vi "TDMS Cleanup.vi"(0 "Logging in":refnum<class "Logging.lvclass">, 1 "Task Selection":T2={"Task Type Select"=enum."Frequency Task", "Input Select Type"=enum."Force Input", "Collect EMG?"=FALSE, "Collect acceleration?"=FALSE, "EMG Rate"=200, "Acceleration Rate"=200} {"Acceleration Rate" min=1 step=1; "EMG Rate" min=1 step=1}, 2 "Task info":T3={"Number of Trials"=1, "Sampling Rate (Hz)"=200, "Trial Duration (s)"=10, "Adjusted MVC (N)"=5.0, "R Phase"=0, "L Phase"=0, "L Pattern"=1, "R Pattern"=1, "Time Between Trials (s)"=5, "Lissajous Speed"=200} {"Lissajous Speed" min=1 max=200; "Time Between Trials (s)" min=1 step=1; "R Pattern" min=1 max=20 step=1; "L Pattern" min=1 max=20 step=1; "L Phase" min=-180 max=180 step=1; "R Phase" min=-180 max=180 step=1; "Adjusted MVC (N)" min=1.0 max=50.0 step=0.10000000149011612; "Trial Duration (s)" min=1 step=1; "Sampling Rate (Hz)" min=1 step=1; "Number of Trials" min=1 step=1}, 5 "TDMS File":path, 7 "Accel TDMS File":refnum<k34>, 9 "Force TDMS File":refnum<k34>, 11 "error in (no error)":errorcluster, 12 "Movement?":bool, 13 "Auto Clust":T1={"Automate?"=FALSE, "Num Parabs"=1, "Patterns Array"=[], "Phase Array"=[]} {"Num Parabs" min=1 step=1}) -> (4 "Logging out":refnum<class "Logging.lvclass">, 15 "error out":errorcluster)   [LabVIEW 2020, in "Logging.lvlib" / "Logging.lvclass"]
uses:
  Logging.lvclass
  C:/Program Files/National Instruments/LabVIEW 2020/vi.lib/ActorFramework/Actor/Actor.lvclass
  Task info df.ctl
  Task selection df.ctl
  Automate df.ctl
  <vilib>/ActorFramework/Actor/Actor.lvclass/Actor.ctl
  <vilib>/ActorFramework/Message Enqueuer/Message Enqueuer.lvclass/Message Enqueuer.ctl
  Logging.lvclass/Logging.ctl
  <vilib>/ActorFramework/Message Enqueuer/Init from Existing Queue.vi
  <vilib>/Utility/file.llb/Read Delimited Spreadsheet (DBL).vi
  <vilib>/ActorFramework/Message Enqueuer/Message Enqueuer.lvclass
  Logging Messages/Convert to Excel Msg/Convert to Excel Msg.lvclass
  <vilib>/ActorFramework/Actor/Actor.lvclass
panel:
  # "Patterns"
  # "Phase"
  # "Left        Right"
  # "Left        Right"
  # "Input Type"
  # "Task Type"
  # "Left Arm"
  # "Right Arm"
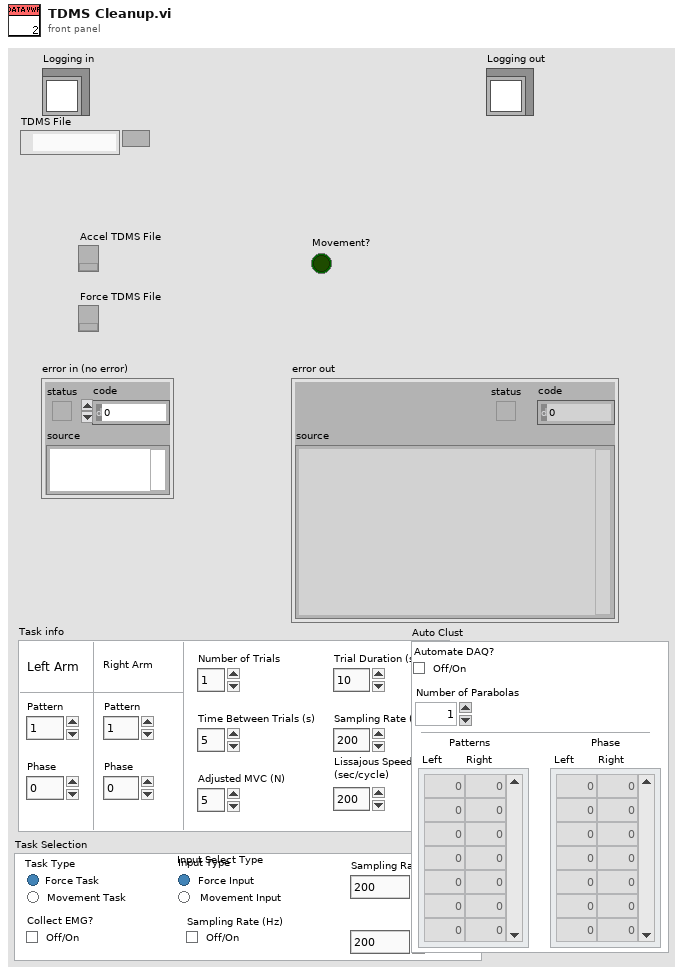
[diagram p1: front panel]
types:
  T1 = typedef "Automate df.ctl" = cluster{"Automate?":bool, "Num Parabs":u16, "Patterns Array":u8[][], "Phase Array":i32[][]}
  T2 = typedef "Task selection df.ctl" = cluster{"Task Type Select":enum32{"Frequency Task", "Scanning Task"}, "Input Select Type":enum32{"Force Input", "Movement Input"}, "Collect EMG?":bool, "Collect acceleration?":bool, "EMG Rate":u16, "Acceleration Rate":u16}
  T3 = typedef "Task info df.ctl" = cluster{"Number of Trials":u8, "Sampling Rate (Hz)":u16, "Trial Duration (s)":u8, "Adjusted MVC (N)":dbl, "R Phase":i32, "L Phase":i32, "L Pattern":u8, "R Pattern":u8, "Time Between Trials (s)":u8, "Lissajous Speed":u16}
  T4 = enum16{"open", "open or create", "create or replace", "create", "open (read-only)"}
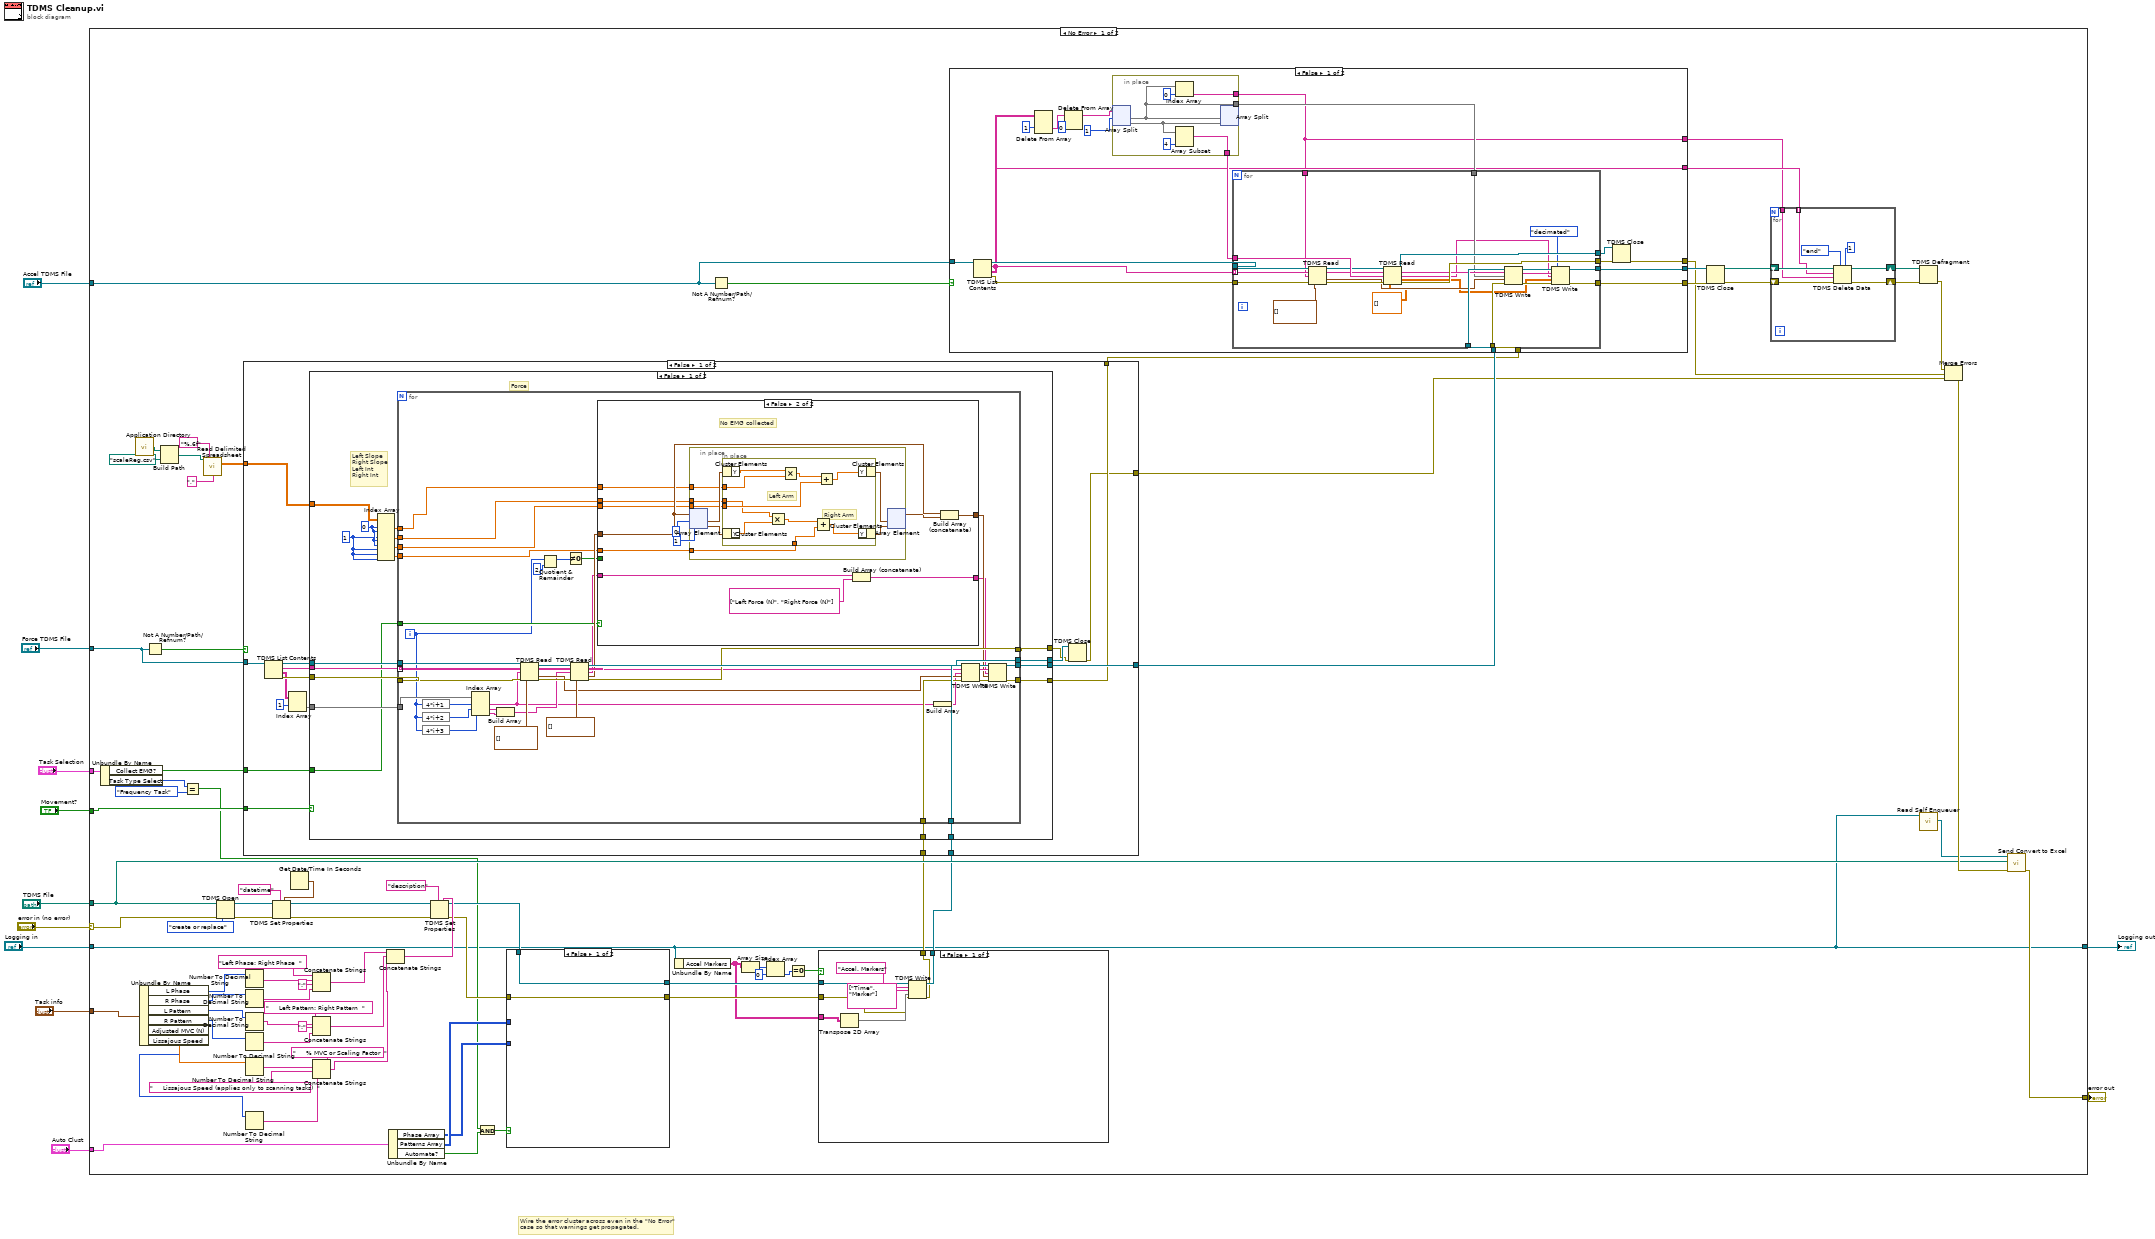
[diagram p0: block diagram]
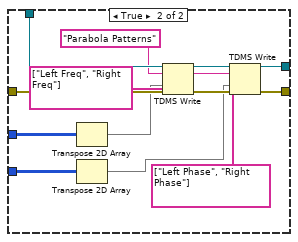
[diagram p3: hidden frame]
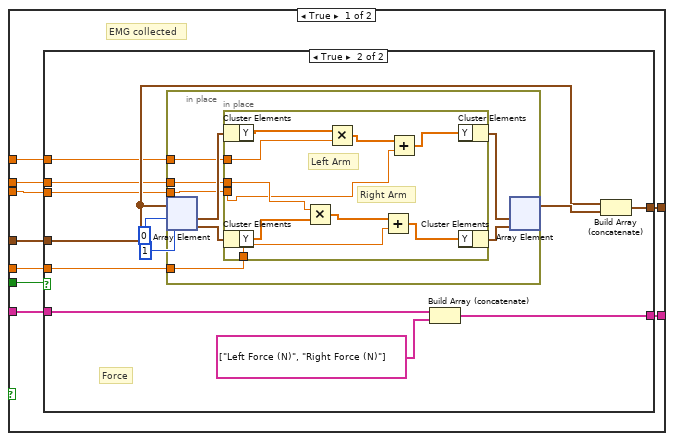
[diagram p4: hidden frame]
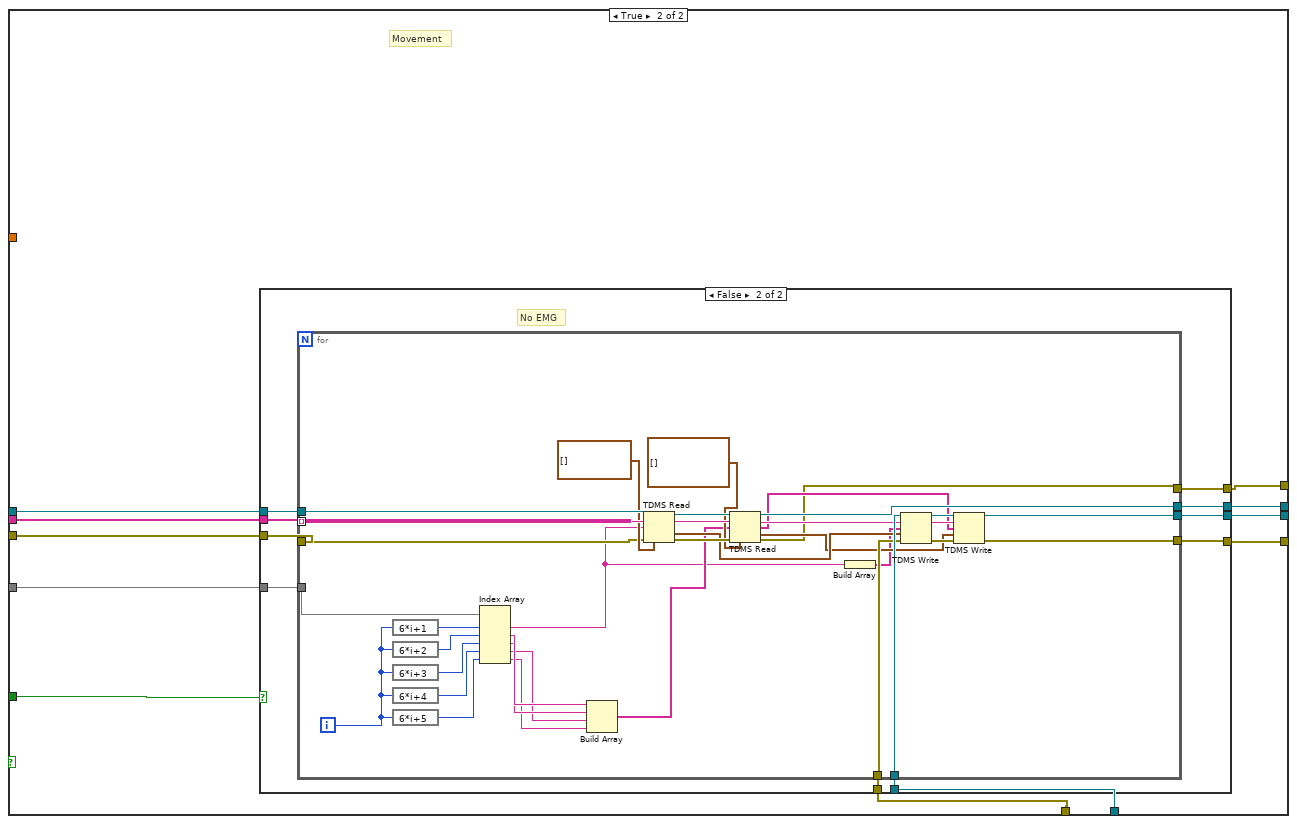
[diagram p6: hidden frame]
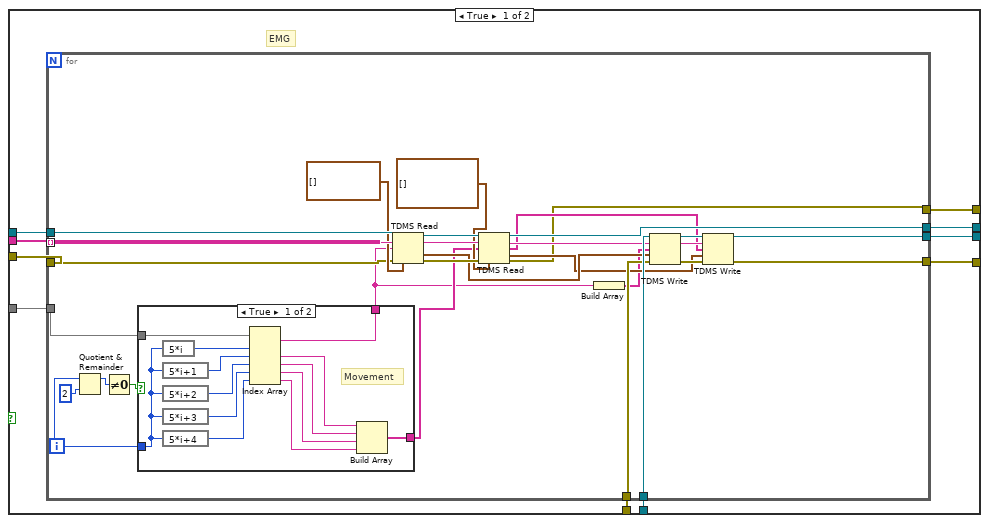
[diagram p7: hidden frame]
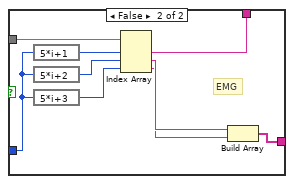
[diagram p8: hidden frame]
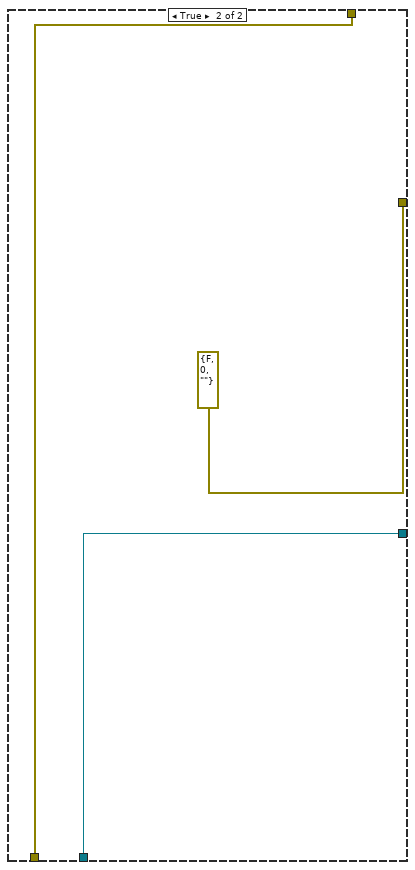
[diagram p9: hidden frame]
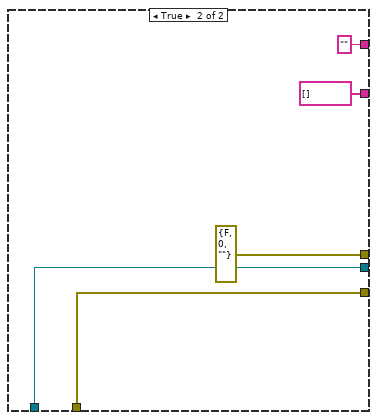
[diagram p10: hidden frame]
diagram:
  # "Wire the error cluster across even in the \"No Error\"\ncase so that warnings get propagated."
  n1 = case shown="No Error" "error in (no error)" {
    selector: "error in (no error)" -> [w82 w452]
    tunnel: [w45 w452] -> w10
    tunnel: [w24 w451] -> w8
    tunnel: "Logging in" -> [w24 w451]
    tunnel: "Accel TDMS File" -> [w85 _]
    tunnel: "Force TDMS File" -> [w86 _]
    tunnel: "TDMS File" -> [w46 _]
    tunnel: "Movement?" -> [w76 _]
    tunnel: "Task Selection" -> [w75 _]
    tunnel: "Task info" -> [w72 _]
    tunnel: "Auto Clust" -> [w43 _]
    frame No Error {
      n2 = Unbundle By Name(w75) -> ("Collect EMG?"=w74:bool, "Task Type Select"=w29:enum32{"Frequency Task", "Scanning Task"})
      n3 = call <vilib>:"Application Directory.vi"() -> ("Application Directory"=w22:path)
      n4 = Unbundle By Name(w72) -> ("L Phase"=w71:i32, "R Phase"=w70:i32, "L Pattern"=w69:u8, "R Pattern"=w68:u8, "Adjusted MVC (N)"=w67:dbl, "Lissajous Speed"=w56:u16)
      n5 = Not A Number/Path/Refnum?(number/path/refnum=w86) -> (NaN/Path/Refnum?=w87:bool)
      n6 = Build Path(base path=w22, name or relative path=path "scaleReg.csv") -> (appended path=w23:path)
      n7 = Equal?(x=w29, y=enum32{"Frequency Task", "Scanning Task"}."Frequency Task") -> (x = y?=w25:bool)
      n8 = call-poly <vilib>:"Read Delimited Spreadsheet.vi"("file path (dialog if empty)"=w23, "format (%.3f)"="%.6f", "delimiter (\\t)"="," ("delimiter (\\t)")) -> ("all rows"=w18:dbl[][])  [unwired: 7 in, 5 out]
      n9 = TDMS Open(8:w82, 10:T4."create or replace" ("operation (0:open)"), 11:w46) -> (0:w91:errorcluster, 3:w92:refnum<k34>)  [unwired: 4 in]
      n10 = Number To Decimal String(number=w71) -> (decimal integer string=w65:string)  [unwired: 1 in]
      n11 = Number To Decimal String(number=w70) -> (decimal integer string=w58:string)  [unwired: 1 in]
      n12 = Number To Decimal String(number=w69) -> (decimal integer string=w64:string)  [unwired: 1 in]
      n13 = Number To Decimal String(number=w68) -> (decimal integer string=w61:string)  [unwired: 1 in]
      n14 = Number To Decimal String(number=w67) -> (decimal integer string=w59:string)  [unwired: 1 in]
      n15 = Number To Decimal String(number=w56) -> (decimal integer string=w55:string)  [unwired: 1 in]
      n16 = Get Date/Time In Seconds() -> (seconds since 1Jan1904=w89:timestamp)
      n17 = TDMS Set Properties(5:w89, 7:"datetime", 8:w91, 11:w92) -> (0:w49:errorcluster, 3:w73:refnum<k34>)  [unwired: 2 in, 2 out]
      n18 = Concatenate Strings("Left Phase: Right Phase  " ("string"), w65, ":" ("string"), w58) -> (w54:string)
      n19 = Concatenate Strings("     Left Pattern: Right Pattern  " ("string"), w64, ":" ("string"), w61) -> (w53:string)
      n20 = Concatenate Strings("     % MVC or Scaling Factor  " ("string"), w59, "     Lissajous Speed (applies only to scanning tasks)  " ("string"), w55) -> (w52:string)
      n21 = Concatenate Strings(w54, w53, w52) -> (w51:string)
      n22 = Unbundle By Name(w43) -> ("Phase Array"=w30:i32[][], "Patterns Array"=w42:u8[][], "Automate?"=w26:bool)
      n23 = TDMS Set Properties(5:w51, 7:"description" ("property names"), 8:w49, 11:w73) -> (0:w40:errorcluster, 3:w41:refnum<k34>)  [unwired: 2 in, 2 out]
      n24 = And(x=w25, y=w26) -> (x .and. y?=w27:bool)
      n25 = case shown="False" w27 {
        tunnel: w42 -> [_ w123]
        tunnel: w41 -> [w113 w127]
        tunnel: w40 -> [w112 w126]
        tunnel: [w113 w121] -> w39
        tunnel: [w112 w119] -> w38
        tunnel: w30 -> [_ w115]
        frame False {
        }
        frame True {
          n26 = Transpose 2D Array(2D array=w123) -> (transposed array=w122:u8[][])
          n27 = Transpose 2D Array(2D array=w115) -> (transposed array=w114:i32[][])
          n28 = TDMS Write(0:w127, 5:"Parabola Patterns" ("group name in (Untitled)"), 7:string[] ["Left Freq", "Right Freq"] ("array"), 9:w122, 11:w126) -> (4:w120:refnum<k34>, 6:w117:string, 15:w118:errorcluster)  [unwired: 1 in, 1 out]
          n29 = TDMS Write(0:w120, 5:w117, 7:string[] ["Left Phase", "Right Phase"] ("channel name(s) in (Untitled)"), 9:w114, 11:w118) -> (4:w121:refnum<k34>, 15:w119:errorcluster)  [unwired: 1 in, 2 out]
        }
      }
      n30 = Unbundle By Name(w24) -> ("Accel Markers"=w31:string[][])
      n31 = Not A Number/Path/Refnum?(number/path/refnum=w85) -> (NaN/Path/Refnum?=w88:bool)
      n32 = Array Size(array=w31) -> (size(s)=w37:i32[])
      n33 = Index Array(array=w37, index=0) -> (element=w35:i32)
      n34 = Equal To 0?(x=w35) -> (x = 0?=w34:bool)
      n35 = case shown="False" w34 {
        tunnel: w39 -> [w109 w111]
        tunnel: w38 -> [w102 w110]
        tunnel: [w106 w111] -> w33
        tunnel: [w105 w110] -> w32
        tunnel: w31 -> [w104 _]
        frame False {
          n36 = Transpose 2D Array(2D array=w104) -> (transposed array=w103:string[][])
          n37 = TDMS Write(0:w109, 5:"Accel. Markers" ("group name in (Untitled)"), 7:string[] ["Time", "Marker"] ("channel name(s) in (Untitled)"), 9:w103, 11:w102) -> (4:w106:refnum<k34>, 15:w105:errorcluster)  [unwired: 1 in, 2 out]
        }
        frame True {
        }
      }
      n38 = case shown="False" w87 {
        tunnel: w86 -> [w144 _]
        tunnel: w33 -> [w142 w394]
        tunnel: [w141 w394] -> w84
        tunnel: w32 -> [w140 w393]
        tunnel: [w139 w393] -> w81
        tunnel: [w138 errorcluster {"status"=FALSE, "code"=0, "source"=""} ("error out")] -> w79
        tunnel: w76 -> [w130 _]
        tunnel: w74 -> [w129 _]
        tunnel: w18 -> [w128 _]
        frame False {
          n39 = TDMS List Contents(7:w144) -> (0:w134:errorcluster, 1:w133:string[][], 2:w137:string[], 3:w143:refnum<k34>)  [unwired: 2 in]
          n40 = Index Array(array=w133, index (row)=1) -> (element=w131:string[])  [unwired: 1 in]
          n41 = case shown="False" w130 {
            tunnel: w143 -> [w162 w285]
            tunnel: w142 -> [w161 w284]
            tunnel: [w160 w283] -> w141
            tunnel: w140 -> [w159 w282]
            tunnel: [w158 w281] -> w139
            tunnel: w137 -> [w157 w280]
            tunnel: [w156 w279] -> w136
            tunnel: [w155 w278] -> w135
            tunnel: w134 -> [w154 w277]
            tunnel: w131 -> [w153 w276]
            tunnel: w129 -> [w152 w275]
            tunnel: w128 -> [w145 _]
            frame False {
              w150 = 1 ("index (row)")
              w151 = 0 ("index (row)")
              # "Left Slope\nRight Slope\nLeft Int\nRight Int"
              # "Force"
              n42 = Index Array(array=w145, index (row) #1=w151, index (col) #1=w151, index (row) #2=w150, index (col) #2=w151, index (row) #3=w151, index (col) #3=w150, index (row) #4=w150, index (col) #4=w150) -> (element #1=w149:dbl, element #2=w147:dbl, element #3=w148:dbl, element #4=w146:dbl)
              n43 = for {
                tunnel: w162 -> [w203]
                tunnel: w157 -> [w202] mode=indexing
                tunnel: w161 -> [w201]
                tunnel: [w193] -> w160
                tunnel: w159 -> [w200]
                tunnel: [w190] -> w158
                tunnel: [w198] -> w156
                tunnel: [w187] -> w155
                tunnel: w154 -> [w186]
                tunnel: w153 -> [w185]
                tunnel: w152 -> [w174]
                tunnel: w149 -> [w166]
                tunnel: w148 -> [w165]
                tunnel: w147 -> [w164]
                tunnel: w146 -> [w163]
                i -> [w173]
                n44 = expression code="4*i+1"(w173) -> (w184:i32)
                n45 = expression code="4*i+2"(w173) -> (w183:i32)
                n46 = expression code="4*i+3"(w173) -> (w182:i32)
                n47 = Index Array(array=w185, index #1=w184, index #2=w183, index #3=w182) -> (element #1=w178:string, element #2=w181:string, element #3=w180:string)
                n48 = Build Array(w181, w180) -> (w179:string[])
                n49 = TDMS Read(0:w203, 5:w202, 7:w178, 11:w186, 12:timestamp[] []) -> (4:w199:refnum<k34>, 6:w197:string, 10:w188:timestamp[], 15:w196:errorcluster)  [unwired: 3 in, 2 out]
                n50 = Quotient & Remainder(x=w173, y=2) -> (x-y*floor(x/y)=w171:i32)  [unwired: 1 out]
                n51 = Not Equal To 0?(x=w171) -> (x != 0?=w170:bool)
                n52 = TDMS Read(0:w199, 5:w197, 7:w179, 11:w196, 12:waveform(dbl)[] [] ("data")) -> (4:w198:refnum<k34>, 6:w167:string, 8:w169:string[], 10:w176:waveform(dbl)[], 15:w187:errorcluster)  [unwired: 3 in, 1 out]
                n53 = case shown="False" w174 {
                  tunnel: w176 -> [w211 w255]
                  tunnel: [w212 w256] -> w175
                  tunnel: w170 -> [w210 _]
                  tunnel: w169 -> [w209 w250]
                  tunnel: [w208 w249] -> w168
                  tunnel: w166 -> [w207 w248]
                  tunnel: w165 -> [w205 w247]
                  tunnel: w164 -> [w206 w246]
                  tunnel: w163 -> [w204 w245]
                  frame True {
                    # "EMG collected"
                    n54 = case shown="True" w210 {
                      tunnel: [w214 w223] -> w212
                      tunnel: w211 -> [w214 w222]
                      tunnel: w209 -> [w213 w221]
                      tunnel: [w213 w219] -> w208
                      tunnel: w207 -> [_ w218]
                      tunnel: w206 -> [_ w217]
                      tunnel: w205 -> [_ w216]
                      tunnel: w204 -> [_ w215]
                      frame False {
                        # "EMG"
                      }
                      frame True {
                        # "Force"
                        n55 = in-place {
                          in-place-border: w218 -> [w230]
                          in-place-border: w217 -> [w229]
                          in-place-border: w216 -> [w228]
                          in-place-border: w215 -> [w227]
                          n56 = in-place-array #1(w222, 0, 1) -> (w234:waveform(dbl), w233:waveform(dbl))
                          n57 = in-place {
                            in-place-border: w230 -> [w238]
                            in-place-border: w229 -> [w237]
                            in-place-border: w228 -> [w236]
                            in-place-border: w227 -> [w235]
                            # "Right Arm"
                            # "Left Arm"
                            n58 = in-place-cluster #2(w234) -> ("Y"=w243:dbl[])
                            n59 = in-place-cluster #3(w233) -> ("Y"=w239:dbl[])
                            n60 = Multiply(x=w237, y=w239) -> (x*y=w241:dbl[])
                            n61 = Multiply(x=w243, y=w238) -> (x*y=w244:dbl[])
                            n62 = Add(x=w241, y=w235) -> (x+y=w240:dbl[])
                            n63 = Add(x=w244, y=w236) -> (x+y=w242:dbl[])
                            n64 = in-place-cluster #2("Y"=w242) -> (w231:waveform(dbl))
                            n65 = in-place-cluster #3("Y"=w240) -> (w232:waveform(dbl))
                          }
                          n66 = in-place-array #1(w231, w232) -> (w224:waveform(dbl)[])  [unwired: 2 out]
                        }
                        n67 = Build Array (concatenate)(w221, string[] ["Left Force (N)", "Right Force (N)"] ("array")) -> (w219:string[])
                        n68 = Build Array (concatenate)(w222, w224) -> (w223:waveform(dbl)[])
                      }
                    }
                  }
                  frame False {
                    # "No EMG collected"
                    n69 = in-place {
                      in-place-border: w248 -> [w260]
                      in-place-border: w247 -> [w259]
                      in-place-border: w246 -> [w258]
                      in-place-border: w245 -> [w257]
                      n70 = in-place-array #4(w255, 0, 1) -> (w264:waveform(dbl), w263:waveform(dbl))
                      n71 = in-place {
                        in-place-border: w260 -> [w268]
                        in-place-border: w259 -> [w267]
                        in-place-border: w258 -> [w266]
                        in-place-border: w257 -> [w265]
                        # "Right Arm"
                        # "Left Arm"
                        n72 = in-place-cluster #5(w264) -> ("Y"=w273:dbl[])
                        n73 = in-place-cluster #6(w263) -> ("Y"=w269:dbl[])
                        n74 = Multiply(x=w266, y=w269) -> (x*y=w271:dbl[])
                        n75 = Multiply(x=w273, y=w268) -> (x*y=w274:dbl[])
                        n76 = Add(x=w271, y=w265) -> (x+y=w270:dbl[])
                        n77 = Add(x=w274, y=w267) -> (x+y=w272:dbl[])
                        n78 = in-place-cluster #5("Y"=w272) -> (w261:waveform(dbl))
                        n79 = in-place-cluster #6("Y"=w270) -> (w262:waveform(dbl))
                      }
                      n80 = in-place-array #4(w261, w262) -> (w252:waveform(dbl)[])  [unwired: 2 out]
                    }
                    n81 = Build Array (concatenate)(w250, string[] ["Left Force (N)", "Right Force (N)"] ("array")) -> (w249:string[])
                    n82 = Build Array (concatenate)(w255, w252) -> (w256:waveform(dbl)[])
                  }
                }
                n83 = Build Array(w178) -> (w177:string[])
                n84 = TDMS Write(0:w201, 5:w167, 7:w177, 9:w188, 11:w200) -> (4:w192:refnum<k34>, 6:w189:string, 15:w191:errorcluster)  [unwired: 1 in, 1 out]
                n85 = TDMS Write(0:w192, 5:w189, 7:w168, 9:w175, 11:w191) -> (4:w193:refnum<k34>, 15:w190:errorcluster)  [unwired: 1 in, 2 out]
              }
            }
            frame True {
              # "Movement"
              n86 = case shown="False" w275 {
                tunnel: w285 -> [w295 w356]
                tunnel: w284 -> [w294 w355]
                tunnel: [w293 w354] -> w283
                tunnel: w282 -> [w292 w353]
                tunnel: [w291 w352] -> w281
                tunnel: w280 -> [w290 w351]
                tunnel: [w289 w350] -> w279
                tunnel: [w288 w349] -> w278
                tunnel: w277 -> [w287 w348]
                tunnel: w276 -> [w286 w347]
                frame True {
                  # "EMG"
                  n87 = for {
                    tunnel: w295 -> [w324]
                    tunnel: w290 -> [w323] mode=indexing
                    tunnel: w294 -> [w322]
                    tunnel: [w314] -> w293
                    tunnel: w292 -> [w321]
                    tunnel: [w311] -> w291
                    tunnel: [w319] -> w289
                    tunnel: [w305] -> w288
                    tunnel: w287 -> [w304]
                    tunnel: w286 -> [w303]
                    i -> [w299]
                    n88 = Quotient & Remainder(x=w299, y=2) -> (x-y*floor(x/y)=w297:i32)  [unwired: 1 out]
                    n89 = Not Equal To 0?(x=w297) -> (x != 0?=w296:bool)
                    n90 = case shown="True" w296 {
                      tunnel: w303 -> [w337 w346]
                      tunnel: [w331 w340] -> w302
                      tunnel: [w330 w339] -> w301
                      tunnel: w299 -> [w329 w338]
                      frame True {
                        # "Movement"
                        n91 = expression code="5*i"(w329) -> (w336:i32)
                        n92 = expression code="5*i+1"(w329) -> (w335:i32)
                        n93 = expression code="5*i+2"(w329) -> (w334:i32)
                        n94 = expression code="5*i+3"(w329) -> (w328:i32)
                        n95 = expression code="5*i+4"(w329) -> (w327:i32)
                        n96 = Index Array(array=w337, index #1=w336, index #2=w335, index #3=w334, index #4=w328, index #5=w327) -> (element #1=w330:string, element #2=w333:string, element #3=w332:string, element #4=w326:string, element #5=w325:string)
                        n97 = Build Array(w333, w332, w326, w325) -> (w331:string[])
                      }
                      frame False {
                        # "EMG"
                        n98 = expression code="5*i+1"(w338) -> (w345:i32)
                        n99 = expression code="5*i+2"(w338) -> (w344:i32)
                        n100 = expression code="5*i+3"(w338) -> (w343:i32)
                        n101 = Index Array(array=w346, index #1=w345, index #2=w344, index #3=w343) -> (element #1=w339:string, element #2=w342:string, element #3=w341:string)
                        n102 = Build Array(w342, w341) -> (w340:string[])
                      }
                    }
                    n103 = TDMS Read(0:w324, 5:w323, 7:w301, 11:w304, 12:timestamp[] []) -> (4:w320:refnum<k34>, 6:w318:string, 10:w307:timestamp[], 15:w317:errorcluster)  [unwired: 3 in, 2 out]
                    n104 = TDMS Read(0:w320, 5:w318, 7:w302, 11:w317, 12:waveform(dbl)[] [] ("data")) -> (4:w319:refnum<k34>, 6:w310:string, 8:w308:string[], 10:w306:waveform(dbl)[], 15:w305:errorcluster)  [unwired: 3 in, 1 out]
                    n105 = Build Array(w301) -> (w300:string[])
                    n106 = TDMS Write(0:w322, 5:w310, 7:w300, 9:w307, 11:w321) -> (4:w313:refnum<k34>, 6:w309:string, 15:w312:errorcluster)  [unwired: 1 in, 1 out]
                    n107 = TDMS Write(0:w313, 5:w309, 7:w308, 9:w306, 11:w312) -> (4:w314:refnum<k34>, 15:w311:errorcluster)  [unwired: 1 in, 2 out]
                  }
                }
                frame False {
                  # "No EMG"
                  n108 = for {
                    tunnel: w356 -> [w391]
                    tunnel: w351 -> [w390] mode=indexing
                    tunnel: w355 -> [w389]
                    tunnel: [w381] -> w354
                    tunnel: w353 -> [w388]
                    tunnel: [w378] -> w352
                    tunnel: [w386] -> w350
                    tunnel: [w372] -> w349
                    tunnel: w348 -> [w371]
                    tunnel: w347 -> [w370]
                    i -> [w361]
                    n109 = expression code="6*i+1"(w361) -> (w369:i32)
                    n110 = expression code="6*i+2"(w361) -> (w368:i32)
                    n111 = expression code="6*i+3"(w361) -> (w367:i32)
                    n112 = expression code="6*i+4"(w361) -> (w360:i32)
                    n113 = expression code="6*i+5"(w361) -> (w359:i32)
                    n114 = Index Array(array=w370, index #1=w369, index #2=w368, index #3=w367, index #4=w360, index #5=w359) -> (element #1=w363:string, element #2=w366:string, element #3=w365:string, element #4=w358:string, element #5=w357:string)
                    n115 = Build Array(w366, w365, w358, w357) -> (w364:string[])
                    n116 = TDMS Read(0:w391, 5:w390, 7:w363, 11:w371, 12:timestamp[] []) -> (4:w387:refnum<k34>, 6:w385:string, 10:w374:timestamp[], 15:w384:errorcluster)  [unwired: 3 in, 2 out]
                    n117 = TDMS Read(0:w387, 5:w385, 7:w364, 11:w384, 12:waveform(dbl)[] [] ("data")) -> (4:w386:refnum<k34>, 6:w377:string, 8:w375:string[], 10:w373:waveform(dbl)[], 15:w372:errorcluster)  [unwired: 3 in, 1 out]
                    n118 = Build Array(w363) -> (w362:string[])
                    n119 = TDMS Write(0:w389, 5:w377, 7:w362, 9:w374, 11:w388) -> (4:w380:refnum<k34>, 6:w376:string, 15:w379:errorcluster)  [unwired: 1 in, 1 out]
                    n120 = TDMS Write(0:w380, 5:w376, 7:w375, 9:w373, 11:w379) -> (4:w381:refnum<k34>, 15:w378:errorcluster)  [unwired: 1 in, 2 out]
                  }
                }
              }
            }
          }
          n121 = TDMS Close(8:w135, 11:w136) -> (0:w138:errorcluster)  [unwired: 1 out]
        }
        frame True {
        }
      }
      n122 = case shown="False" w88 {
        tunnel: w85 -> [w414 _]
        tunnel: w84 -> [w412 w450]
        tunnel: [w411 w450] -> w83
        tunnel: w81 -> [w409 w449]
        tunnel: [w407 w449] -> w80
        tunnel: [w406 errorcluster {"status"=FALSE, "code"=0, "source"=""} ("error out")] -> w78
        tunnel: [w396 string[] [] ("group names")] -> w13
        tunnel: [w395 ""] -> w12
        frame False {
          n123 = TDMS List Contents(7:w414) -> (0:w397:errorcluster, 1:w402:string[][], 2:w396:string[], 3:w413:refnum<k34>)  [unwired: 2 in]
          n124 = Delete From Array(array=w402, index (row)=1) -> (deleted portion=w404:string[])  [unwired: 2 in, 1 out]
          n125 = Delete From Array(array=w404, index=0) -> (array with subset deleted=w401:string[])  [unwired: 1 in, 1 out]
          n126 = in-place {
            in-place-border: [w415] -> w399
            in-place-border: [w419] -> w395
            in-place-border: [w418] -> w398
            n127 = in-place-split #7(w401, 1) -> (w418:string[], w417:string[])
            n128 = Index Array(array=w418, index=0) -> (element=w419:string)
            n129 = Array Subset(array=w417, length=4) -> (w415:string[])  [unwired: 1 in]
            n130 = in-place-split #7(w418, w417) -> ()  [unwired: 2 out]
          }
          n131 = for {
            tunnel: w413 -> [w440]
            tunnel: w396 -> [w438] mode=indexing
            tunnel: w412 -> [w435]
            tunnel: [w445] -> w411
            tunnel: [w444] -> w410
            tunnel: w409 -> [w426]
            tunnel: [w443] -> w408
            tunnel: [w442] -> w407
            tunnel: w399 -> [w441]
            tunnel: w395 -> [w431]
            tunnel: w398 -> [w430]
            tunnel: w397 -> [w422]
            n132 = TDMS Read(0:w440, 5:w438, 7:w431, 11:w422, 12:timestamp[] []) -> (4:w439:refnum<k34>, 6:w437:string, 10:w425:timestamp[], 15:w436:errorcluster)  [unwired: 3 in, 2 out]
            n133 = TDMS Read(0:w439, 5:w437, 7:w441, 11:w436, 12:dbl[][] [] ("subarray")) -> (4:w444:refnum<k34>, 6:w433:string, 8:w428:string[], 10:w423:dbl[][], 15:w443:errorcluster)  [unwired: 3 in, 1 out]
            n134 = TDMS Write(0:w435, 5:w433, 7:w430, 9:w425, 11:w426) -> (4:w434:refnum<k34>, 6:w432:string, 15:w429:errorcluster)  [unwired: 1 in, 1 out]
            n135 = TDMS Write(0:w434, 1:enum16{"decimated", "interleaved"}."decimated" ("data layout (0:decimated)"), 5:w432, 7:w428, 9:w423, 11:w429) -> (4:w445:refnum<k34>, 15:w442:errorcluster)  [unwired: 2 out]
          }
          n136 = TDMS Close(8:w408, 11:w410) -> (0:w406:errorcluster)  [unwired: 1 out]
        }
        frame True {
        }
      }
      n137 = TDMS Close(8:w80, 11:w83) -> (0:w17:errorcluster, 3:w16:path)
      n138 = for {
        shift-right: [w98] -> w14
        shift-left: w17 -> [w101]
        shift-right: [w99] -> w15
        shift-left: w16 -> [w100]
        tunnel: w13 -> [w96] mode=indexing
        tunnel: w12 -> [w95]
        n139 = TDMS Delete Data(5:i64 1 ("count (-1: all)"), 7:enum16{"start", "end"}."end" ("from (0: start)"), 8:w101, 9:w95, 10:w96, 11:w100) -> (0:w98:errorcluster, 3:w99:path)  [unwired: 1 in]
      }
      n140 = call <vilib>:"Read Self Enqueuer.vi"("Actor"=w24) -> ("Self Enqueuer"=w44:refnum<class "Message Enqueuer.lvclass">)  [unwired: 10 in]
      n141 = TDMS Defragment(4:w14, 7:w15) -> (0:w77:errorcluster)
      n142 = Merge Errors(w77, w78, w79) -> (w47:errorcluster)
      n143 = call "Send Convert to Excel.vi"("error in (no error)"=w47, "Path to TDMS/TDM File"=w46, "Message Enqueuer in"=w44) -> ("error out"=w45:errorcluster)  [unwired: 7 in, 1 out]
    }
    frame Error {
    }
  }
  "error out" <- w10
  "Logging out" <- w8
